vi "example.vi"() -> ()   [LabVIEW 2013, in "main.lvlib"]
uses:
  main.lvlib
  Controls/Enum Variables.ctl
panel:
  out "Output 2":string
  in  "Input":string="HALLO"
  out "Output":string
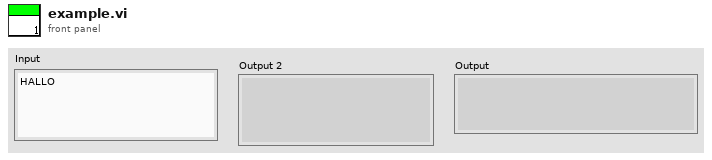
[diagram p1: front panel]
types:
  T1 = typedef "main.lvlib/Enum Variables.ctl" = enum16{"SetAcqFilter", "GetAcqFilter", "Set Filter", "Get Filter", "Set Height", "Get Height", "Set Blue Pressure", "Get Blue Pressure", "Set Red Pressure", "Get Red Pressure", "Init", "Reset Pressure", "Set Red Cursors", "Get Red Cursors", "Set Blue Cursors", "Get Blue Cursors", "Set Language", "Get Language", "Set Active Graphs", "Get ActiveGraphs", "Set Method", "Get Method", "Set Encryption", "Get Encryption", "Set ExcelVersion", "Get ExcelVersion", "Set DICOM Avail", "Get DICOM Avail", "Set DICOM Encode", "Get DICOM Encode", "Set JournalExport", "Get JournalExport", "Set Sequence", "Get Sequence", "Set DAQ Connected", "Get DAQ Connected", "Set Current Graph", "Get Current Graph", "Set General Settings", "Get Hyphenation", "Set Arm Calc Method", "Get Arm Calc Method", "Set Dicom Tags", "Get Dicom Tags", "Set BT Serial", "Get BT Serial", "Set BT Accepted Serials", "Get BT Accepted Serials", "Get BT License", "Set BT License"}
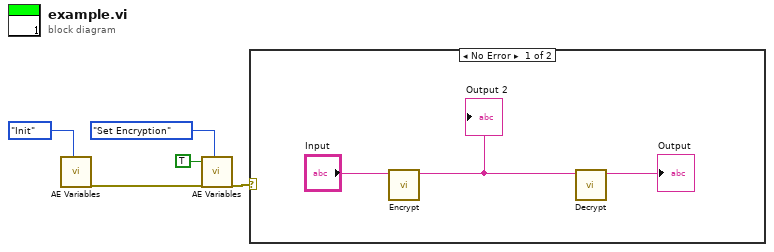
[diagram p0: block diagram]
diagram:
  n1 = call "AE Variables.vi"("Action"=Enum_Variables."Init") -> ("error out"=w3:errorcluster)  [unwired: 11 in, 7 out]
  n2 = call "AE Variables.vi"("VariantIn"=TRUE, "error in (no error)"=w3, "Action"=Enum_Variables."Set Encryption") -> ("error out"=w1:errorcluster)  [unwired: 9 in, 7 out]
  n3 = case shown="No Error" w1 {
    frame No Error {
      n4 = call "Encrypt.vi"("Input"="Input") -> ("Output"=w6:string)  [unwired: 10 in]
      "Output 2" <- w6
      n5 = call "Decrypt.vi"("Input"=w6) -> ("Output"=→"Output":string)  [unwired: 10 in]
    }
    frame Error {
    }
  }
